vi "通信原理实验任务 1_1何德轩.vi"(1 "bits":i32, 2 "decimal":i32) -> (0 "bitstream":i32[](array[numeric]))   [LabVIEW 2018]
panel:
  out "0, 1":i16[](array[numeric])
  out "布尔数组":bool[](array[boolean])
  # "将给定十进制数转换为二进制数，用数组表示并指定数组位数"
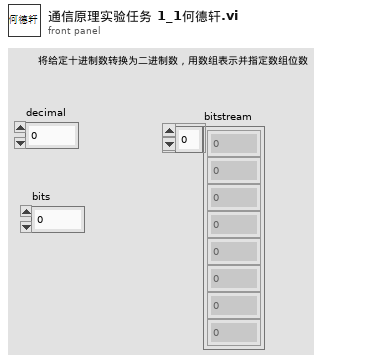
[diagram p1: front panel]
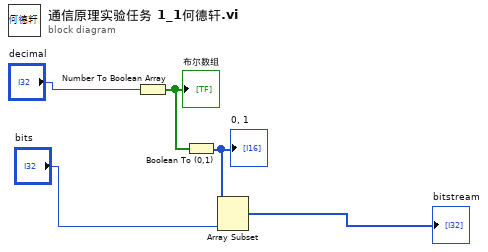
[diagram p0: block diagram]
diagram:
  n1 = Number To Boolean Array(number="decimal") -> (Boolean array=w4:bool[])
  "布尔数组" <- w4
  n2 = Boolean To (0,1)(Boolean=w4) -> (0, 1=w2:i16[])
  "0, 1" <- w2
  n3 = Array Subset(array=w2, length="bits") -> (→"bitstream":i16[])  [unwired: 1 in]
